vi "Config.vi"(8 "error in (no error)":errorcluster, 10 "Setting":variant, 11 "Sim Fgen in":refnum<class "Sim Fgen.lvclass">) -> (0 "error out":errorcluster, 3 "Sim Fgen out":refnum<class "Sim Fgen.lvclass">)   [LabVIEW 2025, in "Fgen.lvlib" / "Sim Fgen.lvclass"]
uses:
  Sim Fgen.lvclass
  Sim Fgen.lvclass/Sim Fgen.ctl
  <vilib>/measure/NI_MABase.lvlib
  Fgen configuration/Fgen configuration.lvclass
  Fgen Channel/Fgen Channel.lvclass
  Fgen Channel configuration/Fgen Channel configuration.lvclass
  Users/Public/Documents/Sandia National Labs/TSS Plugin/Abstract Engine.lvlibp/Abstract Instrument/Channel.ctl
  Users/Public/Documents/Sandia National Labs/TSS Plugin/Abstract Engine.lvlibp/Abstract Instrument/Abstract Instrument.lvclass
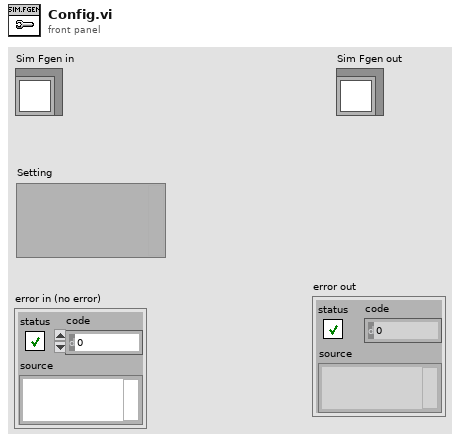
[diagram p1: front panel]
types:
  T1 = typedef "Abstract Engine.lvlibp/Instrument configuration.lvclass/Default Instrument.ctl" = cluster{"Type":string, "Address":string, "SW Alias":string, "Description":string, "Enabled":bool}
  T2 = typedef "Fgen.lvlib/Fgen configuration.lvclass/Fgen Setting.ctl" = cluster{"Type":string, "Output Mode":string, "Sample Rate":dbl, "Samples":dbl, "Gain":dbl, "Trigger":string, "Impedance":string, "Offset":dbl}
  T3 = typedef "Abstract Engine.lvlibp/Abstract Instrument.lvclass/Channel.ctl" = cluster{"Alias":string, "DataType":enum16{"Anaolg Input", "Waveform"}, "Unit":enum16{"---", "V", "A", "Ohm", "Hz", "uF", "degC", "deg"}, "Upper limit":dbl, "Lower limit":dbl, "Measurement":variant}
  T4 = typedef "Fgen.lvlib/Fgen Channel configuration.lvclass/Fgen Channel Setting.ctl" = cluster{"Trgger Type":string, "Duty Cycle":dbl, "Amplitude":dbl, "Frequency":dbl, "Output Shape":string, "Phase":dbl}
  T5 = typedef "Abstract Engine.lvlibp/Channel configuration.lvclass/Default Channel.ctl" = cluster{"Address":string, "SW Alias":string, "Enabled":bool, "Type":string, "Description":string}
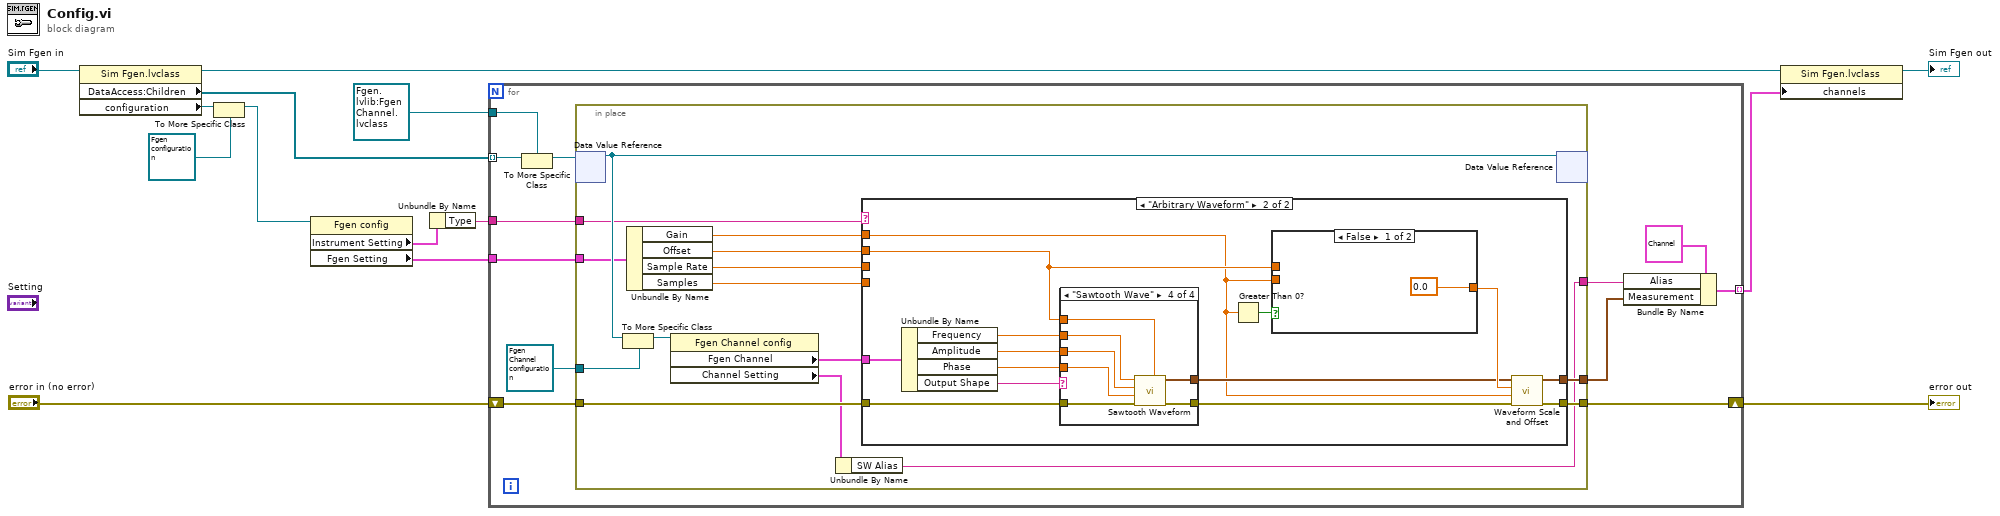
[diagram p0: block diagram]
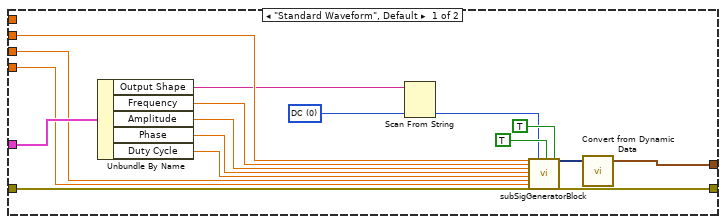
[diagram p2: hidden frame]
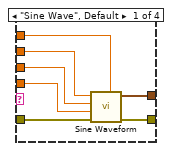
[diagram p3: hidden frame]
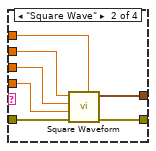
[diagram p4: hidden frame]
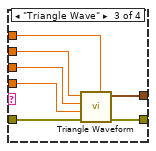
[diagram p5: hidden frame]
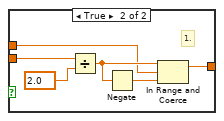
[diagram p6: hidden frame]
diagram:
  n1 = property class="Sim Fgen.lvclass"(reference="Sim Fgen in") -> (reference out=w10:refnum<class "Sim Fgen.lvclass">, "DataAccess:Children"=w6:refnum<data-value>[], "configuration"=w7:refnum<class "CEF_serializable configuration.lvclass">)  [unwired: 1 in, 1 out]
  n2 = To More Specific Class(target class=refnum<class "Fgen configuration.lvclass"> refnum ("Fgen.lvlib:Fgen configuration.lvclass"), reference=w7) -> (specific class reference=w8:refnum<class "Fgen configuration.lvclass">)  [unwired: 1 in, 1 out]
  n3 = property class="Fgen config"(reference=w8) -> ("Instrument Setting"=w4:T1, "Fgen Setting"=w2:T2)  [unwired: 1 in, 2 out]
  n4 = Unbundle By Name(w4) -> ("Type"=w3:string)
  n5 = for {
    shift-right: [w25] -> w11
    shift-left: "error in (no error)" -> [w26]
    tunnel: w6 -> [w24] mode=indexing
    tunnel: refnum<data-value> refnum ("data value reference") -> [w23]
    tunnel: w2 -> [w21]
    tunnel: w3 -> [w19]
    tunnel: [w17] -> w1 mode=indexing
    n6 = To More Specific Class(target class=w23, reference=w24) -> (specific class reference=w22:refnum<data-value>)  [unwired: 1 in, 1 out]
    n7 = in-place {
      in-place-border: w26 -> [w41]
      in-place-border: [w40] -> w25
      in-place-border: [w39] -> w18
      in-place-border: refnum<class "Fgen Channel configuration.lvclass"> refnum ("Fgen.lvlib:Fgen Channel configuration.lvclass") -> [w37]
      in-place-border: w21 -> [w35]
      in-place-border: w19 -> [w30]
      in-place-border: [w27] -> w16
      n8 = in-place-dvr #1(w22) -> (w36:refnum<class "Fgen Channel.lvclass">)  [unwired: 1 out]
      n9 = To More Specific Class(target class=w37, reference=w36) -> (specific class reference=w38:refnum<class "Fgen Channel configuration.lvclass">)  [unwired: 1 in, 1 out]
      n10 = Unbundle By Name(w35) -> ("Gain"=w34:dbl, "Offset"=w33:dbl, "Sample Rate"=w32:dbl, "Samples"=w31:dbl)
      n11 = property class="Fgen Channel config"(reference=w38) -> ("Fgen Channel"=w29:T4, "Channel Setting"=w28:T5)  [unwired: 1 in, 2 out]
      n12 = Unbundle By Name(w28) -> ("SW Alias"=w27:string)
      n13 = case shown="\"Arbitrary Waveform\"" w30 {
        tunnel: w41 -> [w51 w65]
        tunnel: [w50 w69] -> w40
        tunnel: w29 -> [w58 w62]
        tunnel: [w49 w70] -> w39
        tunnel: w34 -> [_ w59]
        tunnel: w33 -> [w48 w60]
        tunnel: w32 -> [w45 _]
        tunnel: w31 -> [w46 _]
        frame "Standard Waveform", Default {
          w43 = u16 0 items=["DC", "Sine", "Square", "Triangle", "Sawtooth"] ("Generate")
          n14 = Unbundle By Name(w58) -> ("Output Shape"=w44:string, "Frequency"=w54:dbl, "Amplitude"=w53:dbl, "Phase"=w52:dbl, "Duty Cycle"=w47:dbl)
          n15 = Scan From String(input string=w44, default 1=w43) -> (output 1=w42:u16)  [unwired: 3 in, 3 out]
          n16 = call <vilib>:"subSigGeneratorBlock.vi"("Offset"=w48, "Frequency"=w54, "Amplitude"=w53, "Phase"=w52, "Duty Cycle (%)"=w47, "Sampling Rate (Hz)"=w45, "# of Samples"=w46, "error in (no error)"=w51, "Generate"=w42, "Generate Data in Real Time"=TRUE, "relative time?"=TRUE) -> ("Signal"=w57:dynamicdata, "error out"=w50:errorcluster)  [unwired: 11 in, 4 out]
          n17 = call "Convert from Dynamic Data"("Dynamic Data Type"=w57) -> ("Waveform"=w49:waveform(dbl))  [unwired: 1 in, 2 out]
        }
        frame "Arbitrary Waveform" {
          n18 = Unbundle By Name(w62) -> ("Frequency"=w66:dbl, "Amplitude"=w67:dbl, "Phase"=w68:dbl, "Output Shape"=w63:string)
          n19 = case shown="\"Sawtooth Wave\"" w63 {
            tunnel: w66 -> [w78 w86 w90 w96]
            tunnel: [w73 w85 w87 w98] -> w61
            tunnel: w67 -> [w77 w84 w89 w95]
            tunnel: w60 -> [w79 w83 w91 w97]
            tunnel: w68 -> [w76 w82 w88 w94]
            tunnel: w65 -> [w75 w81 w93 w100]
            tunnel: [w74 w80 w92 w99] -> w64
            frame "Sine Wave", Default {
              n20 = call <vilib>:"Sine Waveform.vi"("offset"=w79, "error in (no error)"=w75, "phase"=w76, "amplitude"=w77, "frequency"=w78) -> ("error out"=w74:errorcluster, "signal out"=w73:waveform(dbl))  [unwired: 5 in]
            }
            frame "Square Wave" {
              n21 = call <vilib>:"Square Waveform.vi"("offset"=w83, "error in (no error)"=w81, "phase"=w82, "amplitude"=w84, "frequency"=w86) -> ("error out"=w80:errorcluster, "signal out"=w85:waveform(dbl))  [unwired: 5 in]
            }
            frame "Triangle Wave" {
              n22 = call <vilib>:"Triangle Waveform.vi"("offset"=w91, "error in (no error)"=w93, "phase"=w88, "amplitude"=w89, "frequency"=w90) -> ("error out"=w92:errorcluster, "signal out"=w87:waveform(dbl))  [unwired: 5 in]
            }
            frame "Sawtooth Wave" {
              n23 = call <vilib>:"Sawtooth Waveform.vi"("offset"=w97, "error in (no error)"=w100, "phase"=w94, "amplitude"=w95, "frequency"=w96) -> ("error out"=w99:errorcluster, "signal out"=w98:waveform(dbl))  [unwired: 5 in]
            }
          }
          n24 = Greater Than 0?(x=w59) -> (x > 0?=w72:bool)
          n25 = case shown="False" w72 {
            tunnel: w59 -> [_ w106]
            tunnel: [0.0 ("DC Offset") w103] -> w71
            tunnel: w60 -> [_ w102]
            frame False {
            }
            frame True {
              # "1."
              n26 = Divide(x=w106, y=2.0) -> (x/y=w105:dbl)
              n27 = Negate(x=w105) -> (-x=w104:dbl)
              n28 = In Range and Coerce(upper limit=w105, x=w102, lower limit=w104) -> (coerced(x)=w103:dbl)  [unwired: 1 out]
            }
          }
          n29 = call <vilib>:"Waveform Scale and Offset.vi"("error in (no error)"=w64, "scale"=w59, "offset"=w71, "waveform in"=w61) -> ("error out"=w69:errorcluster, "waveform out"=w70:waveform(dbl))  [unwired: 6 in]
        }
      }
      n30 = in-place-dvr #1(w36) -> ()  [unwired: 2 out]
    }
    n31 = Bundle By Name(cluster=T3 {"Alias"="ch0", "DataType"=enum."Anaolg Input", "Unit"=enum."V", "Upper limit"=10.0, "Lower limit"=-10.0, "Measurement"=variant} ("Channel"), "Alias"=w16, "Measurement"=w18) -> (w17:T3)
  }
  "error out" <- w11
  n32 = property class="Sim Fgen.lvclass"(reference=w10, "channels"=w1) -> (reference out=→"Sim Fgen out":refnum<class "Sim Fgen.lvclass">)  [unwired: 1 in, 1 out]
